vi "KE622x -- DCon Mode Set Abort On Comp State.vi"(0 "Resource In":refnum<visa-resource-name>, 1 "Check For SCPI Errors? (T)":bool=TRUE, 7 "Abort On Compliance?":bool, 11 "error in (no error)":errorcluster) -> (4 "Resource Out (dupl)":refnum<visa-resource-name>, 15 "error out":errorcluster)   [LabVIEW 2019, in "Keithley 622x.lvlib"]
uses:
  Keithley 622x.lvlib
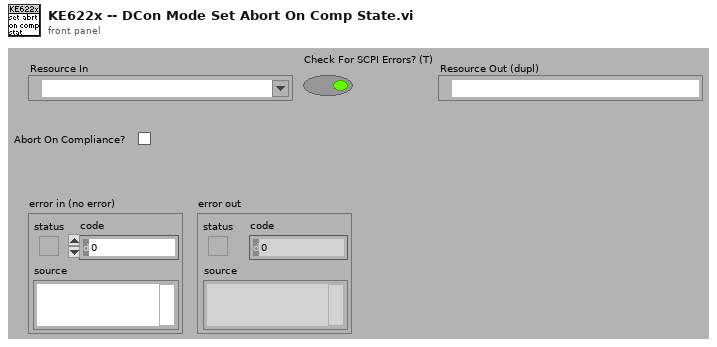
[diagram p1: front panel]
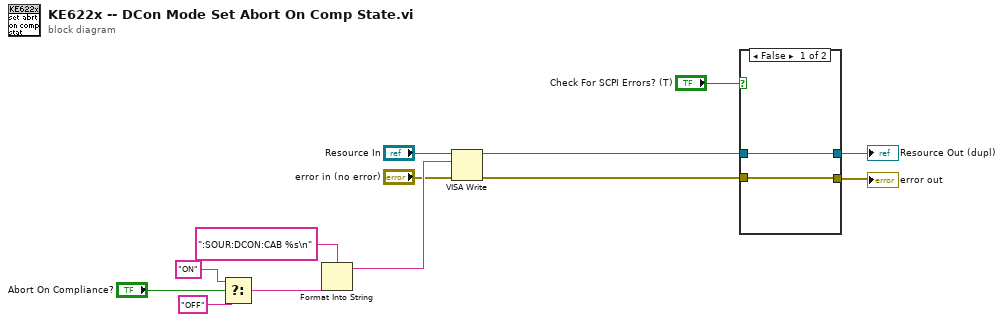
[diagram p0: block diagram]
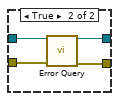
[diagram p2: hidden frame]
diagram:
  n1 = Select(t="ON", s="Abort On Compliance?", f="OFF") -> (s? t:f=w1:string)
  n2 = Format Into String(format string=":SOUR:DCON:CAB %s\n", w1) -> (resulting string=w11:string)  [unwired: 2 in, 1 out]
  n3 = VISA Write(VISA resource name="Resource In", write buffer=w11, error in (no error)="error in (no error)") -> (VISA resource name out=w8:refnum<visa-resource-name>, error out=w7:errorcluster)  [unwired: 1 out]
  n4 = case shown="False" "Check For SCPI Errors? (T)" {
    tunnel: w8 -> [w15 w19]
    tunnel: w7 -> [w14 w18]
    tunnel: [w14 w17] -> w5
    tunnel: [w15 w16] -> w6
    frame False {
    }
    frame True {
      n5 = call "Error Query.vi"("VISA Resource In"=w19, "error in (no error)"=w18) -> ("VISA Resource Out (dupl)"=w16:refnum<visa-resource-name>, "error out"=w17:errorcluster)  [unwired: 10 in, 2 out]
    }
  }
  "Resource Out (dupl)" <- w6
  "error out" <- w5
